vi "ReadFailCount.vi"(7 "ProductModle":string, 8 "error in (no error)":errorcluster, 11 "Statistics path":path) -> (0 "error out":errorcluster, 1 "Fail":u32, 2 "Pass":u32, 3 "file path":path, 4 "yield":dbl, 5 "Total":u32)   [LabVIEW 2019, in "TestBench.lvlib" / "TestBench.lvclass"]
uses:
  TestBench.lvclass
  <vilib>/Utility/config.llb/Read Key (U32).vi
  <vilib>/Utility/config.llb/NI_LVConfig.lvlib
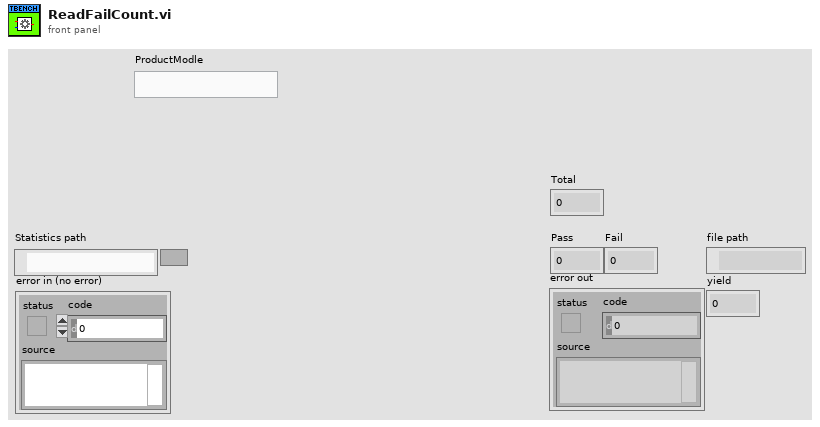
[diagram p1: front panel]
types:
  T1 = typedef "NI_LVConfig.lvlib/Config Data RefNum.ctl" = refnum<k1>
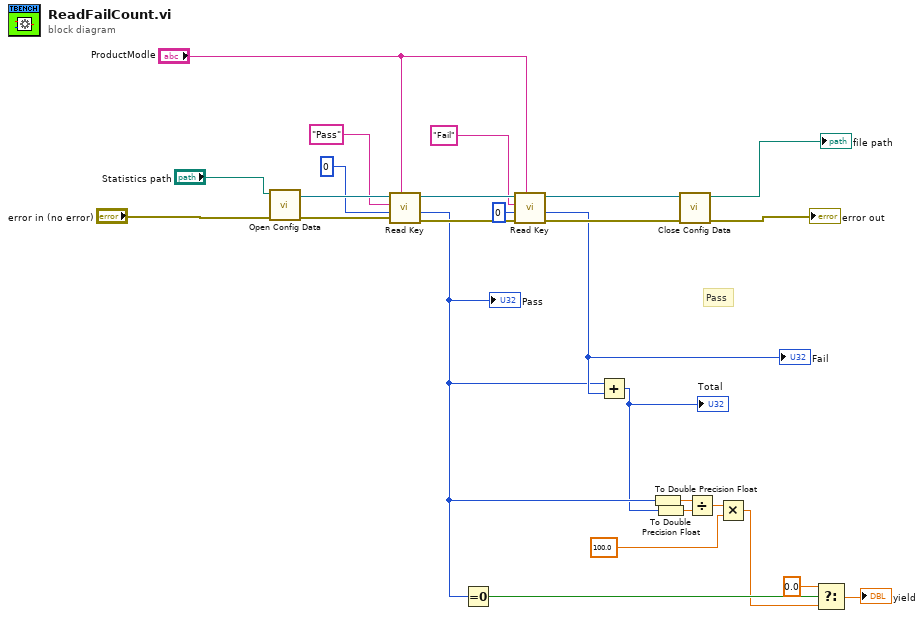
[diagram p0: block diagram]
diagram:
  # "Pass"
  n1 = call <vilib>:"Open Config Data.vi"("error in (no error)"="error in (no error)", "configuration file path"="Statistics path") -> ("error out"=w24:errorcluster, "refnum"=w25:T1)  [unwired: 7 in, 1 out]
  n2 = call-poly <vilib>:"Read Key.vi"("section"="ProductModle", "error in (no error)"=w24, "default value"=u32 0, "key"="Pass", "refnum"=w25) -> ("error out"=w20:errorcluster, "value"=w6:u32, "refnum out"=w21:T1)  [unwired: 3 in, 1 out]
  "Pass" <- w6
  n3 = Equal To 0?(x=w6) -> (x = 0?=w12:bool)
  n4 = call-poly <vilib>:"Read Key.vi"("section"="ProductModle", "error in (no error)"=w20, "default value"=u32 0, "key"="Fail", "refnum"=w21) -> ("error out"=w16:errorcluster, "value"=w8:u32, "refnum out"=w17:T1)  [unwired: 3 in, 1 out]
  "Fail" <- w8
  n5 = Add(x=w6, y=w8) -> (x+y=w5:u32)
  "Total" <- w5
  n6 = To Double Precision Float(number=w6) -> (double precision float=w4:dbl)
  n7 = To Double Precision Float(number=w5) -> (double precision float=w3:dbl)
  n8 = call <vilib>:"Close Config Data.vi"("error in (no error)"=w16, "refnum"=w17) -> ("error out"=→"error out":errorcluster, "file path"=→"file path":path)  [unwired: 8 in]
  n9 = Divide(x=w4, y=w3) -> (x/y=w14:dbl)
  n10 = Multiply(x=w14, y=100.0) -> (x*y=w9:dbl)
  n11 = Select(t=0.0, s=w12, f=w9) -> (s? t:f=→"yield":dbl)
